vi "MarkerSearch.vi"(0 "VISA IN":refnum<visa-resource-name>, 5 "error in":errorcluster) -> (14 "VISA Out":refnum<visa-resource-name>, 19 "error out":errorcluster)   [LabVIEW 2018, in "PNA-X.lvlib"]
doc: "*Critical Note:\nA measurement must be active prior to using the marker functions."
uses:
  PNA-X.lvlib
panel:
  in  "Measurement":string="CH1_S11_1"
  in  "Target Value":dbl format="%_6g"
  in  "Filter Peak":i32=3
  in  "Function":string(combo)="MAX"
  in  "Track ON/OFF":bool=TRUE
  in  "Marker number":i32=1
  in  "Channel":i32=1
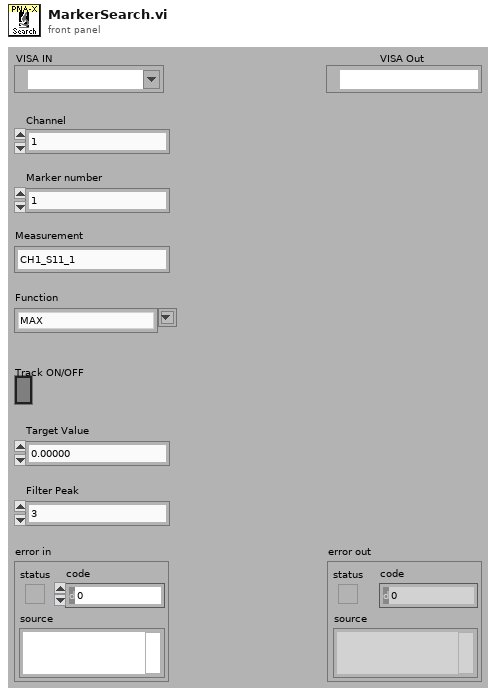
[diagram p1: front panel]
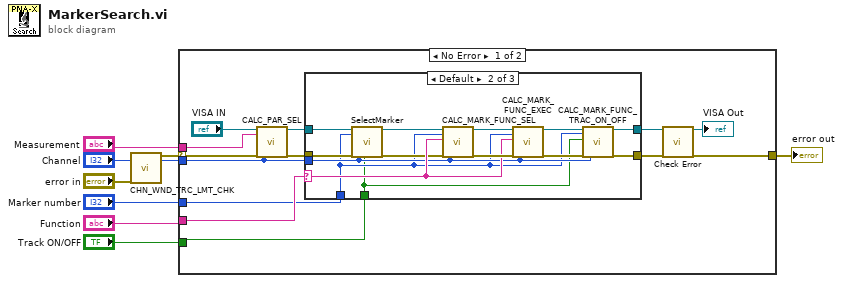
[diagram p0: block diagram]
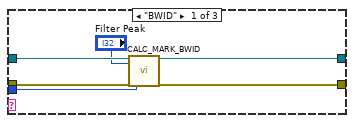
[diagram p2: hidden frame]
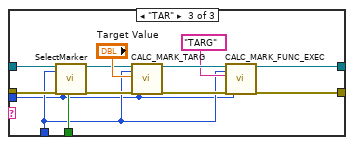
[diagram p3: hidden frame]
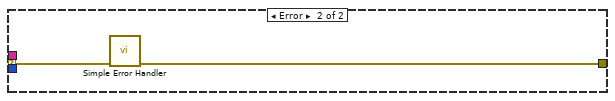
[diagram p4: hidden frame]
diagram:
  n1 = call "CHN_WND_TRC_LMT_CHK.vi"("Channel"="Channel", "error in"="error in") -> ("error out"=w6:errorcluster, "Channel"=w5:i32)  [unwired: 13 in, 3 out]
  n2 = case shown="No Error" w6 {
    selector: w6 -> [w10 w57]
    tunnel: [w22 w56] -> w8
    tunnel: w5 -> [w14 _]
    tunnel: "Marker number" -> [w18 _]
    tunnel: "Function" -> [w20 _]
    tunnel: "Track ON/OFF" -> [w17 _]
    tunnel: "Measurement" -> [w12 _]
    frame No Error {
      n3 = call "CALC_PAR_SEL.vi"("VISA IN"="VISA IN", "Measurement"=w12, "error in"=w10, "Channel"=w14) -> ("VISA Out"=w16:refnum<visa-resource-name>, "error out"=w15:errorcluster)  [unwired: 14 in]
      n4 = case shown="Default" w20 {
        selector: w20 -> [_ w37 _]
        tunnel: w15 -> [w27 w36 w53]
        tunnel: [w26 w40 w47] -> w19
        tunnel: w16 -> [w28 w33 w54]
        tunnel: w14 -> [w25 w34 w44]
        tunnel: w18 -> [_ w31 w45]
        tunnel: w17 -> [_ w30 w52]
        tunnel: [w23 w29 w43] -> w13
        frame "BWID" {
          n5 = call "CALC_MARK_BWID.vi"("VISA IN"=w28, "Filter Peak"="Filter Peak", "error in"=w27, "Channel"=w25) -> ("VISA Out"=w23:refnum<visa-resource-name>, "error out"=w26:errorcluster)  [unwired: 14 in]
        }
        frame Default {
          n6 = call "SelectMarker.vi"("VISA IN"=w33, "Marker"=w31, "error in"=w36, "Channel"=w34, "ON-OFF"=w30) -> ("VISA Out"=w32:refnum<visa-resource-name>, "error out"=w35:errorcluster)  [unwired: 13 in]
          n7 = call "CALC_MARK_FUNC_SEL.vi"("VISA IN"=w32, "Marker number"=w31, "Function"=w37, "error in"=w35, "Channel"=w34) -> ("VISA Out"=w39:refnum<visa-resource-name>, "error out"=w38:errorcluster)  [unwired: 13 in]
          n8 = call "CALC_MARK_FUNC_EXEC.vi"("VISA IN"=w39, "Marker number"=w31, "Function"=w37, "error in"=w38, "Channel"=w34) -> ("VISA Out"=w42:refnum<visa-resource-name>, "error out"=w41:errorcluster)  [unwired: 13 in]
          n9 = call "CALC_MARK_FUNC_TRAC_ON_OFF.vi"("VISA IN"=w42, "Marker number"=w31, "Track ON/OFF"=w30, "error in"=w41, "Channel"=w34) -> ("VISA Out"=w29:refnum<visa-resource-name>, "error out"=w40:errorcluster)  [unwired: 13 in]
        }
        frame "TAR" {
          n10 = call "SelectMarker.vi"("VISA IN"=w54, "Marker"=w45, "error in"=w53, "Channel"=w44, "ON-OFF"=w52) -> ("VISA Out"=w51:refnum<visa-resource-name>, "error out"=w49:errorcluster)  [unwired: 13 in]
          n11 = call "CALC_MARK_TARG.vi"("VISA IN"=w51, "Marker number"=w45, "Target Value"="Target Value", "error in"=w49, "Channel"=w44) -> ("VISA Out"=w50:refnum<visa-resource-name>, "error out"=w48:errorcluster)  [unwired: 13 in]
          n12 = call "CALC_MARK_FUNC_EXEC.vi"("VISA IN"=w50, "Marker number"=w45, "Function"="TARG", "error in"=w48, "Channel"=w44) -> ("VISA Out"=w43:refnum<visa-resource-name>, "error out"=w47:errorcluster)  [unwired: 13 in]
        }
      }
      n13 = call "Check Error.vi"("VISA Resource Name"=w13, "error in (no error)"=w19) -> ("dup VISA session"=→"VISA Out":refnum<visa-resource-name>, "error out"=w22:errorcluster)  [unwired: 16 in]
    }
    frame Error {
      n14 = call <vilib>:"Simple Error Handler.vi"("error in (no error)"=w57) -> ("error out"=w56:errorcluster)  [unwired: 4 in, 4 out]
    }
  }
  "error out" <- w8
